vi "get camera temperature - subvi.vi"(0 "Cooling Status In":T1) -> (1 "Cooling Status Out":T1, 2 "Error?":bool, 3 "temperature out":i32)   [LabVIEW 2014]
uses:
  ctt's/Control 4.ctl
  ctt's/temperature defaults.ctl
  ctt's/Control 2.ctl
  ctt's/Control 3.ctl
  lib/Andorlib/atmcd32d.lvlib
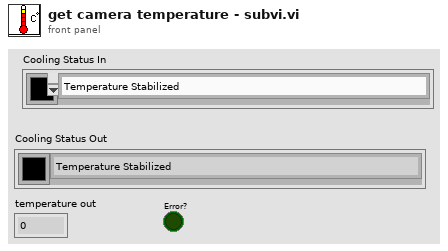
[diagram p1: front panel]
types:
  T1 = cluster{"Color Box":u32, "Cooling Status":enum16{"Temperature Stabilized", "Waiting to Stabilize Temperature", "Cooling is Turned Off", "Have not yet Reached Set Temperature"}}
  T2 = enum16{"Temperature Stabilized", "Waiting to Stabilize Temperature", "Cooling is Turned Off", "Have not yet Reached Set Temperature"}
  T3 = typedef "Control 4.ctl" = u32
  T4 = enum16{"Temperature Stabilized", "Waiting to Stabilize Temperature", "Cooling is Turned Off"}
  T5 = typedef "temperature defaults.ctl" = u32
  T6 = typedef "Control 2.ctl" = u32
  T7 = typedef "Control 3.ctl" = u32
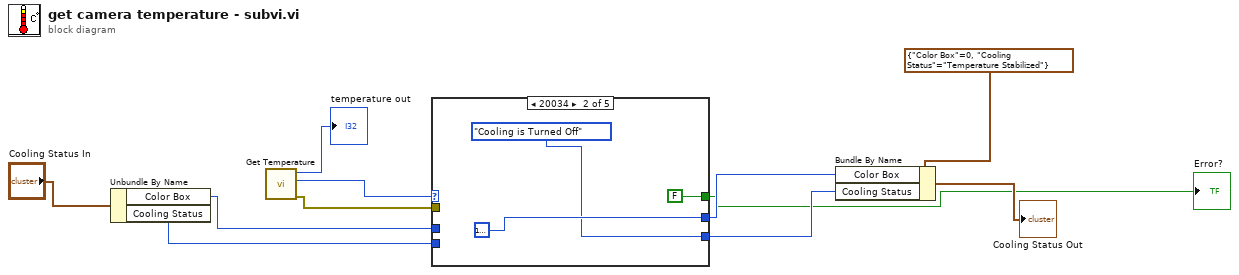
[diagram p0: block diagram]
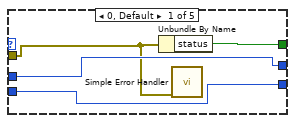
[diagram p2: hidden frame]
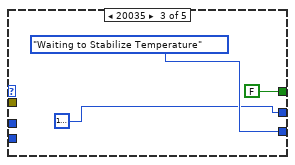
[diagram p3: hidden frame]
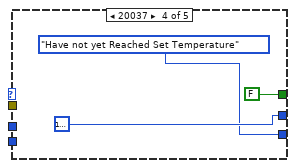
[diagram p4: hidden frame]
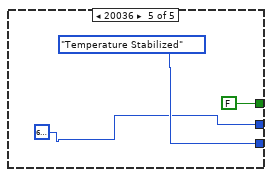
[diagram p5: hidden frame]
diagram:
  n1 = Unbundle By Name("Cooling Status In") -> ("Color Box"=w9:u32, "Cooling Status"=w8:T2)
  n2 = call "Get Temperature.vi"() -> ("error out"=w7:errorcluster, "function return"=w2:u32, "temperature out"=→"temperature out":i32)  [unwired: 9 in]
  n3 = case shown="20034" w2 {
    tunnel: [w15 FALSE ("status") FALSE ("status") FALSE ("status") FALSE ("status")] -> w3
    tunnel: [w14 T3 16711680 T5 16775978 T6 16775978 T7 6618880] -> w6
    tunnel: [w13 T4."Cooling is Turned Off" ("Cooling Status") T4."Waiting to Stabilize Temperature" ("Cooling Status") T2."Have not yet Reached Set Temperature" ("Cooling Status") T4."Temperature Stabilized" ("Cooling Status")] -> w5
    tunnel: w9 -> [w14 _ _ _ _]
    tunnel: w8 -> [w13 _ _ _ _]
    tunnel: w7 -> [w12 _ _ _ _]
    frame 0, Default {
      n4 = Unbundle By Name(w12) -> ("status"=w15:bool)
      n5 = call <vilib>:"Simple Error Handler.vi"("error in (no error)"=w12) -> ()  [unwired: 1 in, 8 out]
    }
    frame 20034 {
    }
    frame 20035 {
    }
    frame 20037 {
    }
    frame 20036 {
    }
  }
  "Error?" <- w3
  n6 = Bundle By Name(cluster=T1 {"Color Box"=0, "Cooling Status"=enum."Temperature Stabilized"} ("Cooling status"), "Color Box"=w6, "Cooling Status"=w5) -> (→"Cooling Status Out":T1)
